vi "Get LakeShore 370 Resistance and Quadrature.vi"(8 "error in":errorcluster, 10 "Channel":i32=1, 11 "VISA resource name":refnum<visa-resource-name>) -> (0 "error out":errorcluster, 1 "Q":dbl, 2 "R":dbl, 3 "VISA resource name out":refnum<visa-resource-name>)   [LabVIEW 2021]
uses:
  GPIB/VISA  Send Receive.vi
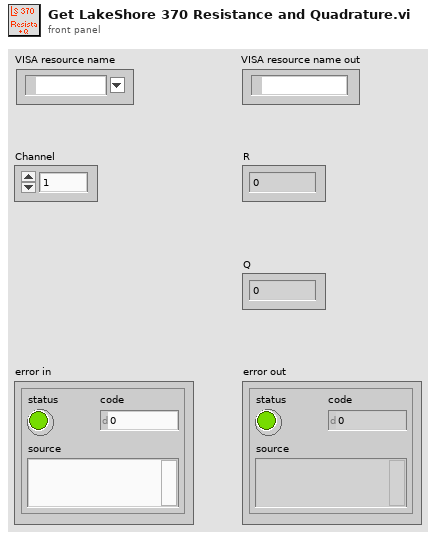
[diagram p1: front panel]
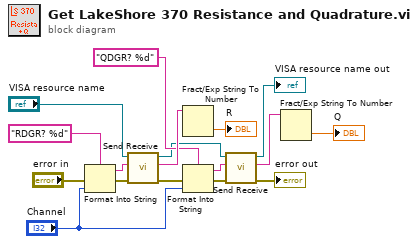
[diagram p0: block diagram]
diagram:
  n1 = Format Into String(format string="RDGR? %d" ("data string in"), error in="error in", "Channel") -> (resulting string=w13:string, error out=w14:errorcluster)  [unwired: 1 in]
  n2 = call-poly "Send Receive.vi"("error in (no error)"=w14, "data string in"=w13, "VISA Resource Name"="VISA resource name") -> ("error out"=w12:errorcluster, "data string out"=w17:string, "VISA Resource Name Out"=w2:refnum<visa-resource-name>)  [unwired: 6 in]
  n3 = Fract/Exp String To Number(string=w17) -> (number=→"R":dbl)  [unwired: 4 out]
  n4 = Format Into String(format string="QDGR? %d" ("data string in"), error in=w12, "Channel") -> (resulting string=w8:string, error out=w11:errorcluster)  [unwired: 1 in]
  n5 = call-poly "Send Receive.vi"("error in (no error)"=w11, "data string in"=w8, "VISA Resource Name"=w2) -> ("error out"=→"error out":errorcluster, "data string out"=w7:string, "VISA Resource Name Out"=→"VISA resource name out":refnum<visa-resource-name>)  [unwired: 6 in]
  n6 = Fract/Exp String To Number(string=w7) -> (number=→"Q":dbl)  [unwired: 4 out]
